vi "Create Mini Explorer.vi"(8 "error in (no error)":errorcluster, 11 "DSF Confguration Session":refnum<class "Configuration Session.lvclass">) -> (0 "error out":errorcluster, 3 "explorer data":T1)   [LabVIEW 2017, in "DSF Mini Explorer.lvlib"]
uses:
  DSF Mini Explorer.lvlib
  VeriStand/Data Sharing Custom Device/Source/DSF Core.lvlibp/Classes/Configuration/Configuration Session.lvclass
  Main VI/Application Data.ctl
  Main VI/View Mode.ctl
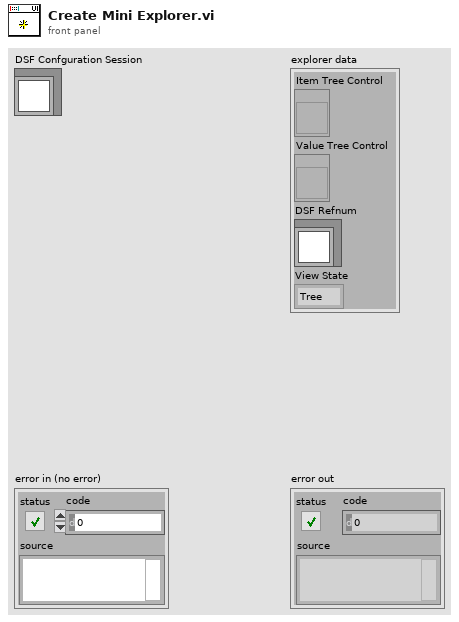
[diagram p1: front panel]
types:
  T1 = typedef "DSF Mini Explorer.lvlib/Application Data.ctl" = cluster{"Item Tree Control":refnum<vi>, "Value Tree Control":refnum<vi>, "DSF Refnum":refnum<class "Configuration Session.lvclass">, "View State":T2}
  T2 = typedef "DSF Mini Explorer.lvlib/View Mode.ctl" = enum16{"Tree", "List"}
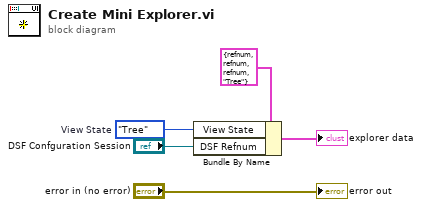
[diagram p0: block diagram]
diagram:
  w4 = View_Mode."Tree"  # View State
  n1 = Bundle By Name(cluster=T1 {"Item Tree Control"=refnum, "Value Tree Control"=refnum, "DSF Refnum"=refnum, "View State"=enum."Tree"}, "View State"=w4, "DSF Refnum"="DSF Confguration Session") -> (→"explorer data":T1)
  "error out" <- "error in (no error)"
